vi "GOOP_HelpMain.vi"(10 "File":string) -> ()   [LabVIEW 2012]
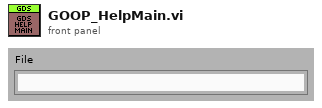
[diagram p1: front panel]
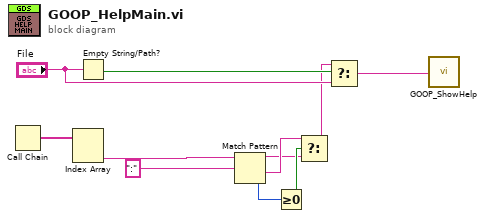
[diagram p0: block diagram]
diagram:
  n1 = Call Chain() -> (call chain=w11:string[])
  n2 = Index Array(array=w11) -> (element #2=w10:string)  [unwired: 2 in, 1 out]
  n3 = Empty String/Path?(string/path="File") -> (empty?=w4:bool)
  n4 = Match Pattern(string=w10, regular expression=":") -> (before substring=w5:string, after substring=w6:string, offset past match=w8:i32)  [unwired: 1 in, 1 out]
  n5 = Greater Or Equal To 0?(x=w8) -> (x >= 0?=w7:bool)
  n6 = Select(t=w6, s=w7, f=w5) -> (s? t:f=w2:string)
  n7 = Select(t=w2, s=w4, f="File") -> (s? t:f=w1:string)
  n8 = call <resource>:"GOOP_ShowHelp.vi"("File"=w1) -> ()
